vi "Initialize.vi"(8 "error in (no error)":errorcluster, 11 "[V] Login in":refnum<class "[V] Login.lvclass">) -> (0 "error out":errorcluster, 3 "[V] Login out":refnum<class "[V] Login.lvclass">)   [LabVIEW 2020, in "[V] Login.lvlib" / "[V] Login.lvclass"]
uses:
  [V] Login.lvclass
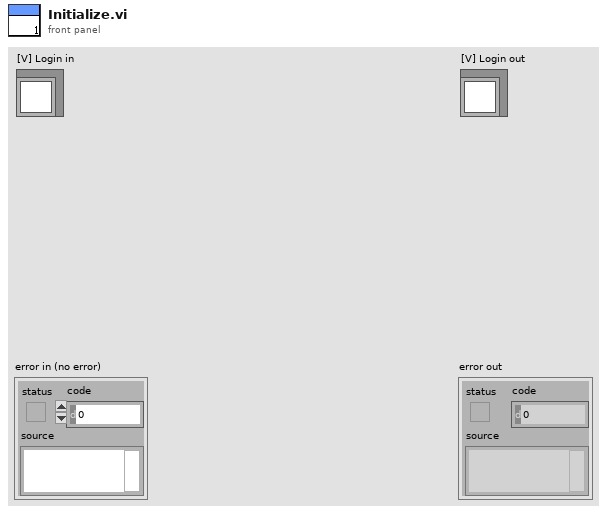
[diagram p1: front panel]
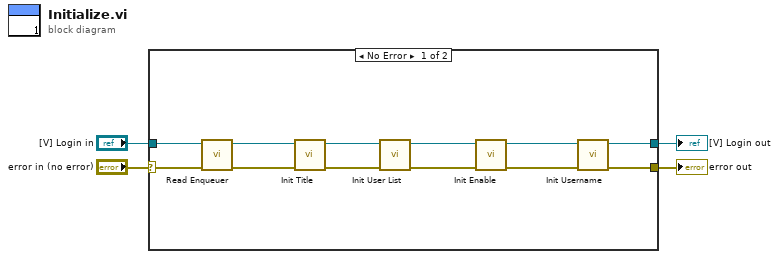
[diagram p0: block diagram]
diagram:
  n1 = case shown="No Error" "error in (no error)" {
    selector: "error in (no error)" -> [w16 w18]
    tunnel: [w7 w18] -> w3
    tunnel: [w8 w17] -> w1
    tunnel: "[V] Login in" -> [w15 w17]
    frame No Error {
      n2 = call "Read Enqueuer.vi"("error in (no error)"=w16, "[V] Login in"=w15) -> ("error out"=w12:errorcluster, "[V] Login out"=w11:refnum<class "[V] Login.lvclass">)  [unwired: 8 in]
      n3 = call "Init Title.vi"("error in (no error)"=w12, "[V] Login in"=w11) -> ("error out"=w6:errorcluster, "[V] Login out"=w5:refnum<class "[V] Login.lvclass">)  [unwired: 8 in]
      n4 = call "Init User List.vi"("error in (no error)"=w6, "[V] Login in"=w5) -> ("error out"=w14:errorcluster, "[V] Login out"=w13:refnum<class "[V] Login.lvclass">)  [unwired: 8 in]
      n5 = call "Init Enable.vi"("error in (no error)"=w14, "[V] Login in"=w13) -> ("error out"=w10:errorcluster, "[V] Login out"=w9:refnum<class "[V] Login.lvclass">)  [unwired: 8 in]
      n6 = call "Init Username.vi"("error in (no error)"=w10, "[V] Login in"=w9) -> ("error out"=w7:errorcluster, "[V] Login out"=w8:refnum<class "[V] Login.lvclass">)  [unwired: 8 in]
    }
    frame Error {
    }
  }
  "error out" <- w3
  "[V] Login out" <- w1
